vi "markers.vi"(11 "project-param in":T1) -> (3 "delimited string":string)   [LabVIEW 2019]
uses:
  Project Parameters.ctl
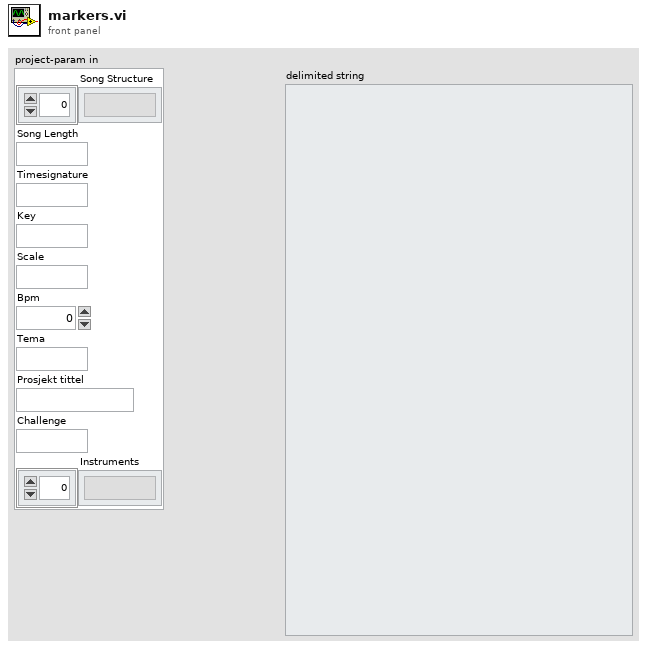
[diagram p1: front panel]
types:
  T1 = typedef "Project Parameters.ctl" = cluster{"Song Structure":string[], "Song Length":string, "Timesignature":string, "Key":string, "Scale":string, "Bpm":i32, "Tema":string, "Prosjekt tittel":string, "Challenge":string, "Instruments":string[]}
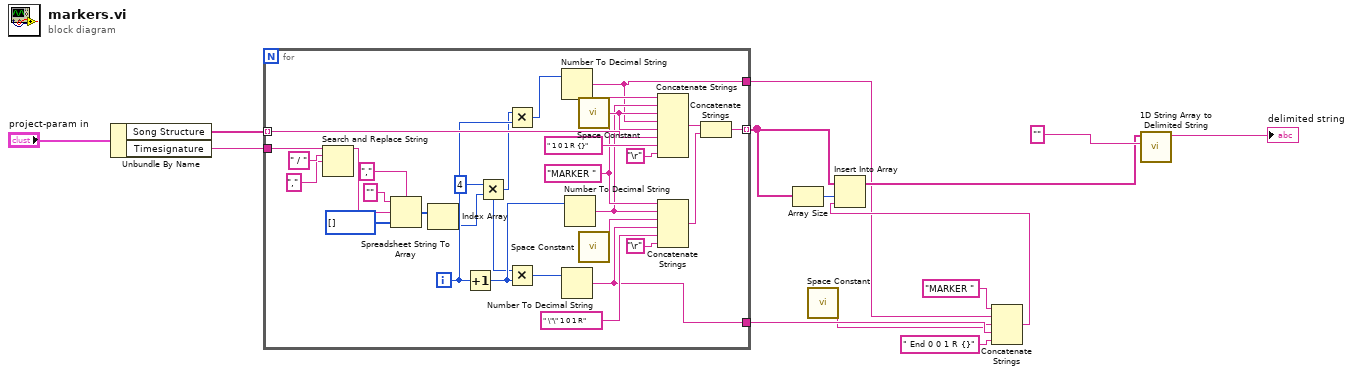
[diagram p0: block diagram]
diagram:
  n1 = Unbundle By Name("project-param in") -> ("Song Structure"=w11:string[], "Timesignature"=w10:string)
  n2 = for {
    tunnel: w11 -> [w42] mode=indexing
    tunnel: w10 -> [w31]
    tunnel: [w32] -> w8 mode=indexing
    tunnel: [w19] -> w3
    tunnel: [w18] -> w2
    i -> [w25]
    w39 = "MARKER "
    n3 = Search and Replace String(input string=w31, search string=" / ", replace string="," ("replace string (\"\")")) -> (result string=w28:string)  [unwired: 5 in, 3 out]
    n4 = Spreadsheet String To Array(delimiter (Tab)=",", format string="", spreadsheet string=w28, array type (2D Dbl)=i32[] []) -> (array=w27:i32[])
    n5 = Index Array(array=w27) -> (element=w17:i32)  [unwired: 1 in]
    n6 = Increment(x=w25) -> (x+1=w22:i32)
    n7 = Multiply(x=4, y=w17) -> (x*y=w15:i32)
    n8 = Multiply(x=w15, y=w25) -> (x*y=w24:i32)
    n9 = Multiply(x=w15, y=w22) -> (x*y=w23:i32)
    n10 = Number To Decimal String(number=w24) -> (decimal integer string=w18:string)  [unwired: 1 in]
    n11 = Number To Decimal String(number=w23) -> (decimal integer string=w19:string)  [unwired: 1 in]
    n12 = Number To Decimal String(number=w22) -> (decimal integer string=w38:string)  [unwired: 1 in]
    n13 = call <vilib>:"Space Constant.vi"() -> ("String"=w43:string)
    n14 = call <vilib>:"Space Constant.vi"() -> ("String"=w37:string)
    n15 = Concatenate Strings(w39, w38, w43, w18, w43, w42, " 1 0 1 R {}" ("string"), "\r") -> (w34:string)
    n16 = Concatenate Strings(w39, w38, w37, w19, " \"\" 1 0 1 R" ("string"), "\r") -> (w33:string)
    n17 = Concatenate Strings(w34, w33) -> (w32:string)
  }
  n18 = Array Size(array=w8) -> (size(s)=w6:i32)
  n19 = call <vilib>:"Space Constant.vi"() -> ("String"=w1:string)
  n20 = Concatenate Strings("MARKER ", w2, w1, w3, " End 0 0 1 R {}") -> (w4:string)
  n21 = Insert Into Array(array=w8, index=w6, new element=w4) -> (w9:string[])
  n22 = call <vilib>:"1D String Array to Delimited String.vi"("delimiter"="", "string array"=w9) -> ("delimited string"=→"delimited string":string)  [unwired: 9 in]
